vi "spring - delete item.vi"(8 "error in (no error)":errorcluster, 10 "Tag (\"\" all)":string, 11 "RefNum in":refnum<vi>) -> (0 "error out":errorcluster, 3 "dup RefNum":refnum<vi>)   [LabVIEW 2014]
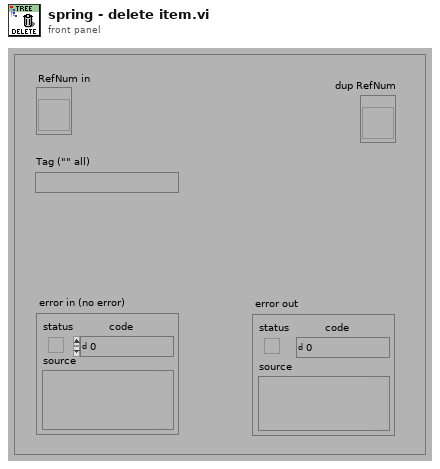
[diagram p1: front panel]
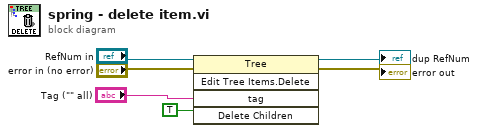
[diagram p0: block diagram]
diagram:
  n1 = invoke class="Tree" method="Edit Tree Items.Delete"(reference="RefNum in", error in="error in (no error)", "tag"="Tag (\"\" all)", "Delete Children"=TRUE) -> (reference out=→"dup RefNum":refnum<vi>, error out=→"error out":errorcluster)  [unwired: 1 in, 3 out]
